vi "DeleteDC.vi"(11 "element":dbl[](array[numeric])) -> (3 "Array":dbl[](array[numeric]))   [LabVIEW 2019]
uses:
  <vilib>/Analysis/baseanly.llb/Mean (DBL).vi
  <vilib>/Analysis/NI_AALBase.lvlib
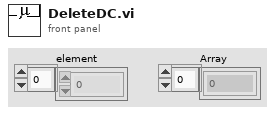
[diagram p1: front panel]
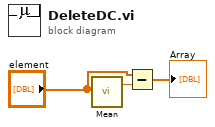
[diagram p0: block diagram]
diagram:
  n1 = call-poly <vilib>:"Mean.vi"("X"="element") -> ("mean"=w1:dbl)  [unwired: 1 out]
  n2 = Subtract(x="element", y=w1) -> (x-y=→"Array":dbl[])
